vi "Add_Pressure_tapping_Info.vi"() -> (5 "Plug in titles":string[](array[string]), 7 "Plug in values":string[](array[string]))   [LabVIEW 2010]
uses:
  Globals/Meas_global.vi
  Globals/Trav_pos_global.vi
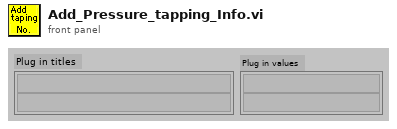
[diagram p1: front panel]
types:
  T1 = typedef "Traverse_cluster.ctl" = cluster{"Start X":dbl, "Start Y":dbl, "Start Z":dbl, "End X":dbl, "End Y":dbl, "End Z":dbl, "No. of pts.":i32, "Spacing":T2, "Filename":path, "Tunnel Speed":dbl, "Averaging time (min)":dbl, "Extra Commands":string, "Specific Arguments":string, "Emission Rate (l/min)":dbl, "Trace Gas Concentration (%)":dbl, "Density Ratio":string, "Comments":string, "Row No":i32, "Row Type Selector":T3, "Completion time":string, "Row Duration (mins)":dbl, "No. of Valid pts.":i32, "Meas Setup File":string}
  T2 = typedef "Spacing.ctl" = enum16{"Linear", "Log", "Gauss", "Specified", "N/A"}
  T3 = typedef "Multi_run_mode.ctl" = enum16{"Move Traverse Only", "Set Tunnel Speed Only", "Set Source Only", "Set Measurement Conditions", "Single Measurement", "Vertical Profile", "Lateral Profile", "Longitudinal Profile", "Explore Volume", "Multi-Axis Profile", "Auto Calibrate", "Meas Fast FID Bkgnd", "Check Beam Power", "Scanning Valve Measurement", "Run VI Named:", "Set ADAM Ch", "Wait (minutes)", "Send Message", "Synchronize With:", "Fall Back to this Row", "Turn Off Row Repeating", "Blank Row"}
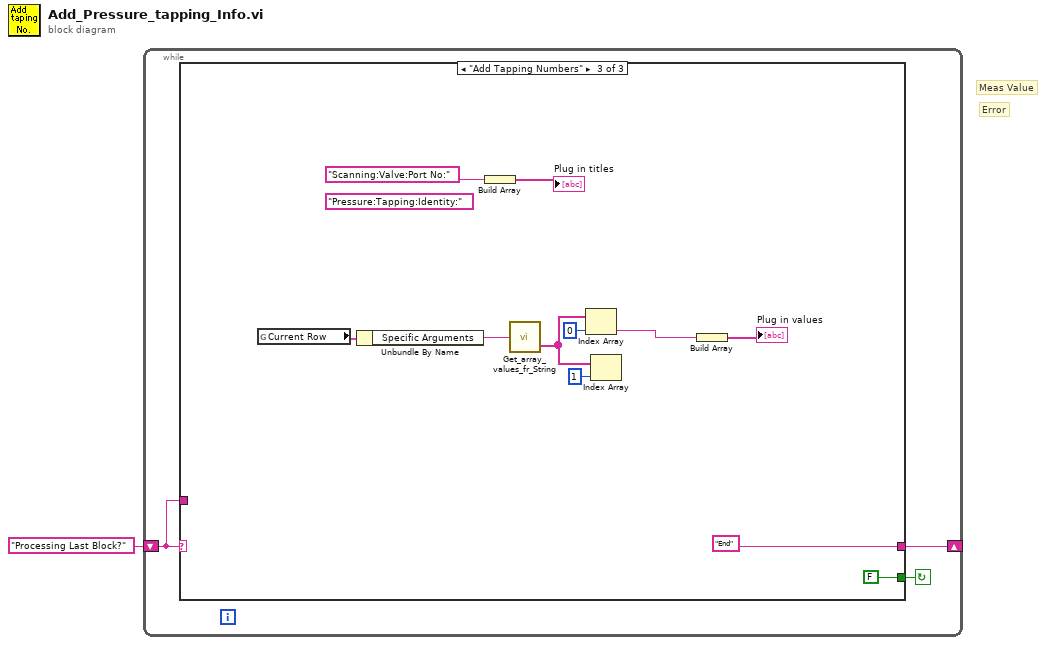
[diagram p0: block diagram]
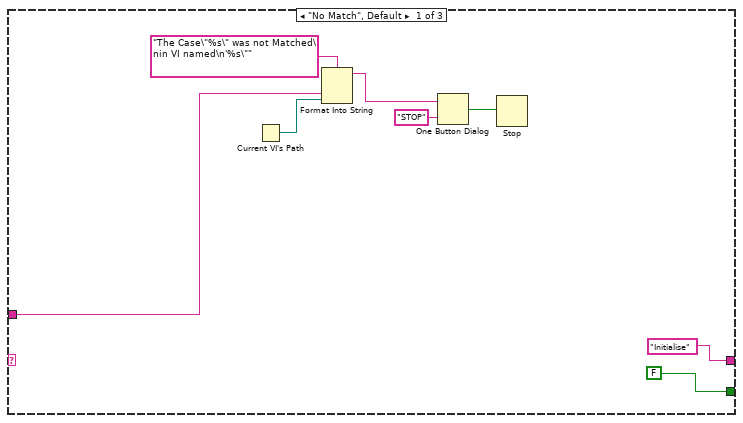
[diagram p2: hidden frame]
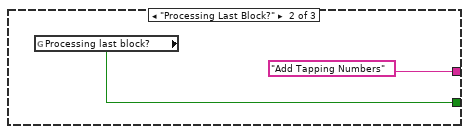
[diagram p3: hidden frame]
diagram:
  # "Error"
  # "Meas Value"
  n1 = while {
    shift-left: "Processing Last Block?" -> [w2]
    shift-right: [w3] -> _
    stop <- w4 continue-if-true
    n2 = case shown="\"Add Tapping Numbers\"" w2 {
      tunnel: [FALSE w13 FALSE ("Processing last block?")] -> w4
      tunnel: ["Initialise" "Add Tapping Numbers" "End"] -> w3
      tunnel: w2 -> [w7 _ _]
      frame "No Match", Default {
        n3 = Current VI's Path() -> (path=w6:path)
        n4 = Format Into String(format string="The Case\"%s\" was not Matched\nin VI named\n'%s\"" ("Format String"), w7, w6) -> (resulting string=w10:string)  [unwired: 2 in, 1 out]
        n5 = One Button Dialog(message=w10, button name ("OK")="STOP") -> (true=w8:bool)
        n6 = Stop(stop? (T)=w8) -> ()
      }
      frame "Processing Last Block?" {
        n7 = global read "Meas_global.vi" "Processing last block?"() -> (w13:bool)
      }
      frame "Add Tapping Numbers" {
        (unwired) "Pressure:Tapping:Identity:"
        n8 = global read "Trav_pos_global.vi" "Current Row"() -> (w23:T1)
        n9 = Unbundle By Name(w23) -> ("Specific Arguments"=w21:string)
        n10 = Build Array("Scanning:Valve:Port No:") -> (→"Plug in titles":string[])
        n11 = call "Get_array_values_fr_String.vi"("String Value"=w21) -> ("String array"=w17:string[])  [unwired: 1 out]
        n12 = Index Array(array=w17, index=0) -> (element=w16:string)
        n13 = Index Array(array=w17, index=1) -> ()  [unwired: 1 out]
        n14 = Build Array(w16) -> (→"Plug in values":string[])
      }
    }
  }
